vi "Facade 1.vi"(0 "Data In":T4, 2 "Display State In":T2, 3 "Container State":T3) -> (6 "Data Out":T4, 7 "Display State Out":T2, 8 "Action":T1)   [LabVIEW 2011, in "StackXControl.xctl"]
uses:
  StackXControl.xctl
  Data 1.ctl
  F:/Program Files (x86)/National Instruments/LabVIEW 2011/examples/lvoop/FriendshipCommunityScope/Stack/Stack.lvclass
  <vilib>/_xctls/Container State.ctl
  State 1.ctl
  <vilib>/_xctls/Action.ctl
  <vilib>/_xctls/XControlSupport.lvlib
panel:
  in  "Stack Contents":dbl[](array[numeric])
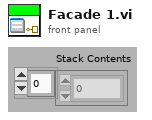
[diagram p1: front panel]
types:
  T1 = typedef "XControlSupport.lvlib/Action.ctl" = cluster{"Data Changed?":bool, "State Changed?":bool, "Action Name":string}
  T2 = typedef "StackXControl.xctl/State 1.ctl" = cluster{"Numeric":dbl}
  T3 = typedef "XControlSupport.lvlib/Container State.ctl" = cluster{"Indicator?":bool, "Run Mode?":bool, " Refnum":refnum<vi>}
  T4 = typedef "StackXControl.xctl/Data 1.ctl" = refnum<class "Stack.lvclass">
  T5 = enum8{"Enabled", "Disabled", "Disabled and Grayed Out"}
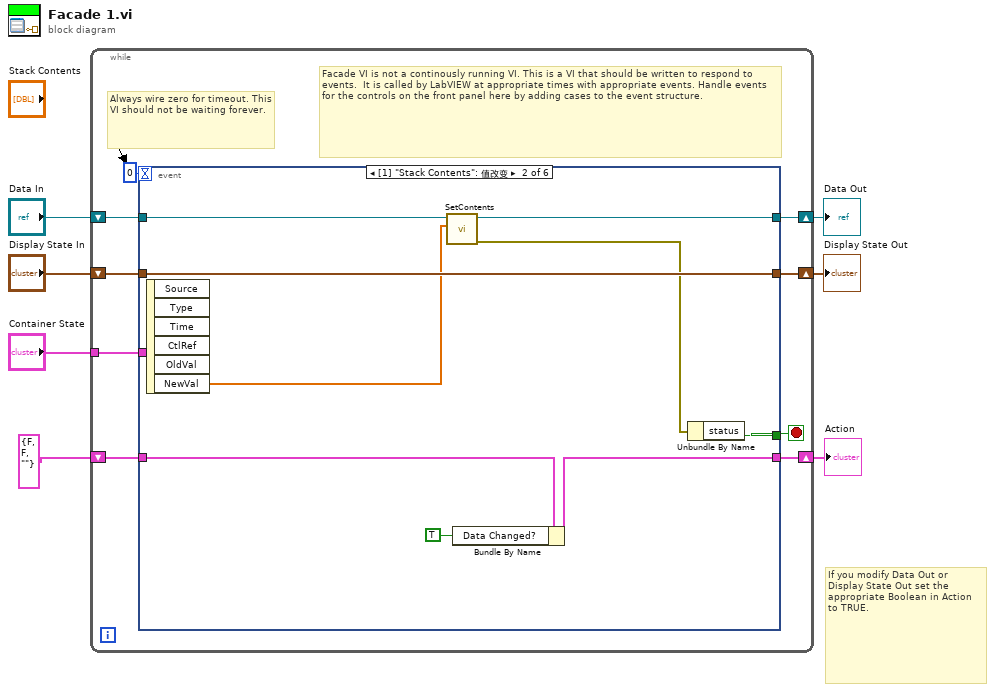
[diagram p0: block diagram]
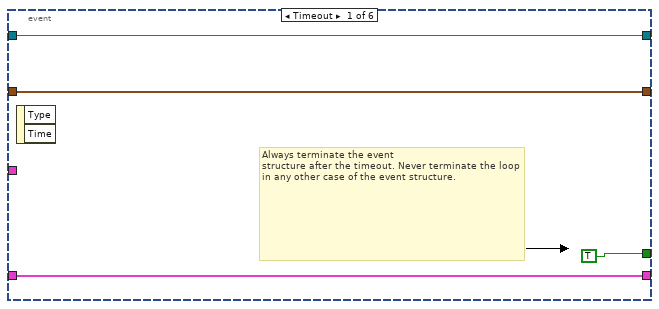
[diagram p2: hidden frame]
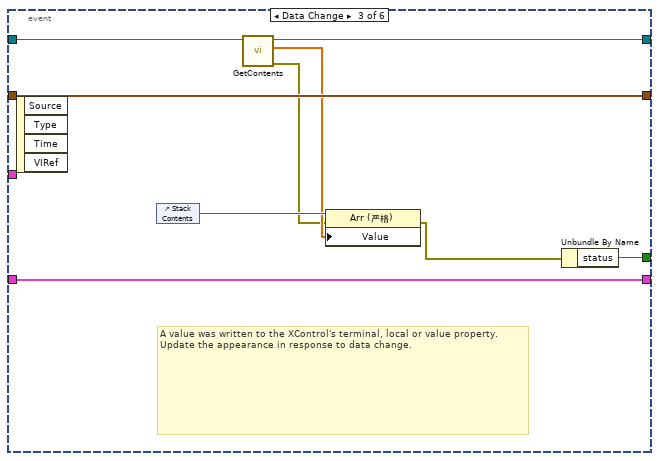
[diagram p3: hidden frame]
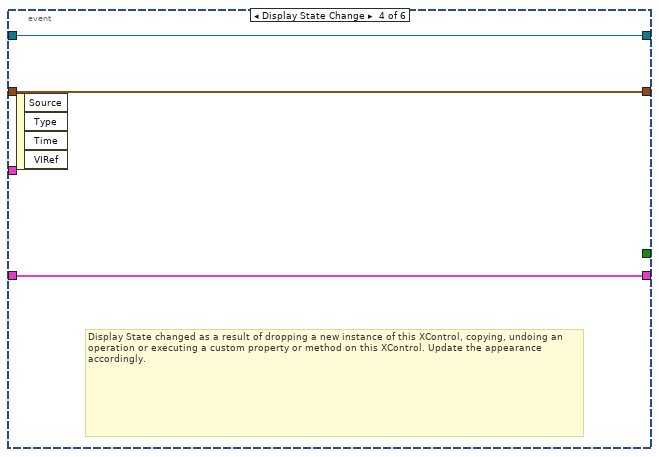
[diagram p4: hidden frame]
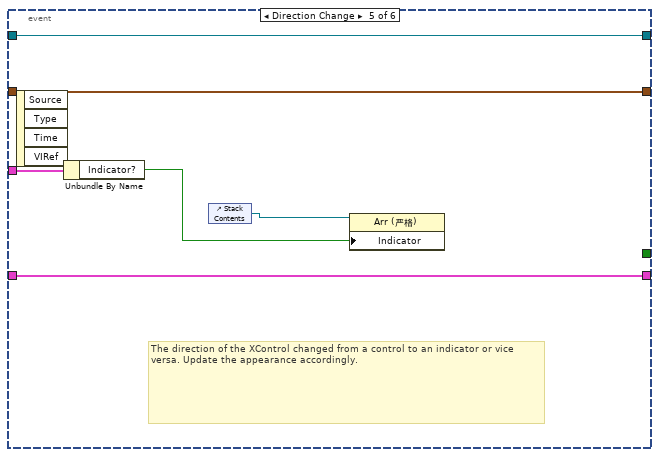
[diagram p5: hidden frame]
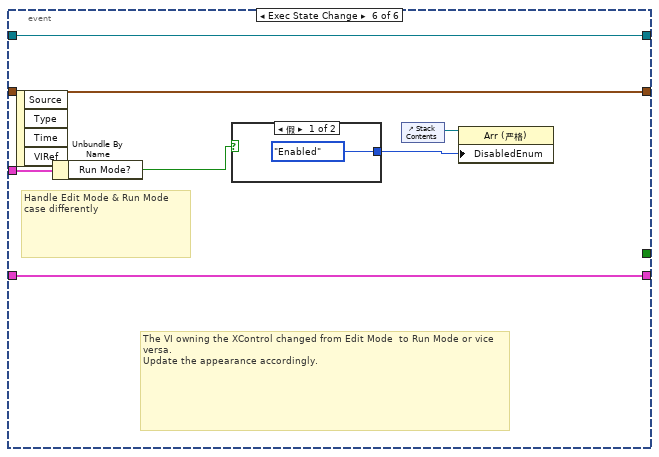
[diagram p6: hidden frame]
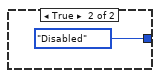
[diagram p7: hidden frame]
diagram:
  # "If you modify Data Out or\nDisplay State Out set the\nappropriate Boolean in Action\nto TRUE."
  n1 = while {
    shift-right: [w15] -> w4
    shift-left: "Display State In" -> [w16]
    tunnel: "Container State" -> [w12]
    shift-right: [w10] -> w7
    shift-left: "Data In" -> [w11]
    shift-right: [w8] -> w2
    shift-left: T1 {"Data Changed?"=FALSE, "State Changed?"=FALSE, "Action Name"=""} ("Action") -> [w9]
    stop <- w14 stop-if-true
    # "Facade VI is not a continously running VI. This is a VI that should be written to respond to events.  It is called by LabVIEW at appropriate times with appropriate events. Handle events for the controls on the front panel here by adding cases to the event structure."
    # "Always wire zero for timeout. This\nVI should not be waiting forever."
    n2 = event shown="[1] \"Stack Contents\": 值改变" {
      selector: _ -> [_ _ _ _ _ _]
      dyn-events: _ -> [_ _ _ _ _ _]
      timeout: 0 -> [_ _ _ _ _ _]
      tunnel: w16 -> [w18 w29 w38 w41 w46 w53]
      tunnel: [w18 w29 w38 w41 w46 w53] -> w15
      tunnel: [TRUE w26 w35 _ _ _] -> w14
      tunnel: w12 -> [_ _ _ _ w47 w54]
      tunnel: w11 -> [w17 w28 w37 w40 w45 w52]
      tunnel: [w17 w27 w36 w40 w45 w52] -> w10
      tunnel: [w19 w22 w30 w39 w44 w51] -> w8
      tunnel: w9 -> [w19 w23 w30 w39 w44 w51]
      event Timeout {
        # "Always terminate the event\nstructure after the timeout. Never terminate the loop in any other case of the event structure."
        n3 = event-data() -> ()  [unwired: 1 in, 2 out]
      }
      event "Stack Contents": Value Change {
        n4 = event-data() -> ("NewVal"=w24:dbl[])  [unwired: 1 in, 5 out]
        n5 = call "SetContents.vi"("Array"=w24, "Stack in"=w28) -> ("error out"=w25:errorcluster, "Stack out"=w27:T4)  [unwired: 8 in]
        n6 = Bundle By Name(cluster=w23, "Data Changed?"=TRUE) -> (w22:T1)
        n7 = Unbundle By Name(w25) -> ("status"=w26:bool)
      }
      event Data Change {
        # "A value was written to the XControl's terminal, local or value property.\nUpdate the appearance in response to data change."
        n8 = event-data() -> ()  [unwired: 1 in, 4 out]
        n9 = control-ref of="Stack Contents"() -> (w34:refnum<vi>)
        n10 = call "GetContents.vi"("Stack in"=w37) -> ("error out"=w32:errorcluster, "Array"=w33:dbl[], "Stack out"=w36:T4)  [unwired: 8 in]
        n11 = property class="Arr (严格)"(reference=w34, error in=w32, "Value"=w33) -> (error out=w31:errorcluster)  [unwired: 1 out]
        n12 = Unbundle By Name(w31) -> ("status"=w35:bool)
      }
      event Display State Change {
        # "Display State changed as a result of dropping a new instance of this XControl, copying, undoing an operation or executing a custom property or method on this XControl. Update the appearance accordingly."
        n13 = event-data() -> ()  [unwired: 1 in, 4 out]
      }
      event Direction Change {
        # "The direction of the XControl changed from a control to an indicator or vice versa. Update the appearance accordingly."
        n14 = event-data() -> ()  [unwired: 1 in, 4 out]
        n15 = Unbundle By Name(w47) -> ("Indicator?"=w42:bool)
        n16 = control-ref of="Stack Contents"() -> (w43:refnum<vi>)
        n17 = property class="Arr (严格)"(reference=w43, "Indicator"=w42) -> ()  [unwired: 1 in, 2 out]
      }
      event Exec State Change {
        # "The VI owning the XControl changed from Edit Mode  to Run Mode or vice versa.\nUpdate the appearance accordingly."
        # "Handle Edit Mode & Run Mode\ncase differently"
        n18 = event-data() -> ()  [unwired: 1 in, 4 out]
        n19 = Unbundle By Name(w54) -> ("Run Mode?"=w48:bool)
        n20 = case shown="假" w48 {
          tunnel: [T5."Enabled" ("Disabled") T5."Disabled" ("Disabled")] -> w49
          frame False {
          }
          frame True {
          }
        }
        n21 = control-ref of="Stack Contents"() -> (w50:refnum<vi>)
        n22 = property class="Arr (严格)"(reference=w50, "DisabledEnum"=w49) -> ()  [unwired: 1 in, 2 out]
      }
    }
  }
  "Display State Out" <- w4
  "Data Out" <- w7
  "Action" <- w2
